vi "test_conv5.vi"() -> ()   [LabVIEW 2018]
uses:
  <vilib>/addons/Modulation/Digital/Channel Coding/MT Convolutional Encoder (Rate).vi
  <vilib>/addons/Modulation/Analog/support/mod_Set Error Source.vi
  <vilib>/addons/Modulation/Digital/Support/Common/Validators/mod_Validate Bit Stream.vi
  <vilib>/addons/Modulation/Digital/Channel Coding/Convolutional codes/mod_Convolutional encoder.vi
  <vilib>/addons/Modulation/Digital/Support/Common/Validators/mod_AWGN Validate.vi
  <vilib>/addons/Modulation/Digital/Impairments/subVIs/mod_createSeeds.vi
  <vilib>/addons/Modulation/Digital/Channel Coding/Convolutional codes/subVIs/mod_Generate encoder tap connections.vi
  <vilib>/addons/Modulation/Digital/Channel Coding/Convolutional codes/subVIs/mod_Perform convolutional encoding.vi
  <vilib>/addons/Modulation/Digital/Channel Coding/Block codes/subVIs/mod_Buffer block code info (I8).vi
  <vilib>/addons/Modulation/Digital/Channel Coding/Convolutional codes/subVIs/mod_Generate valid reset (convolutional, I8).vi
  <vilib>/addons/Modulation/Digital/Support/Common/Validators/mod_Validate Samples Per Symbol.vi
  <vilib>/addons/Modulation/Analog/support/Validators/mod_Validate Complex Waveform.vi
  <vilib>/addons/Modulation/Analog/support/Validators/mod_WFErrorHandler.vi
  <vilib>/addons/Modulation/Digital/Channel Coding/Convolutional codes/subVIs/mod_Select known generator matrix.vi
  <vilib>/addons/Modulation/Digital/Support/Common/Validators/mod_Validate Convolutional Encoder prms.vi
  <vilib>/addons/Modulation/Digital/Support/Common/Validators/mod_Generate Filter Coefficients Validate.vi
  <vilib>/addons/Modulation/Digital/General/subVIs/mod_Generate Filter Coefficients.vi
  <vilib>/addons/Modulation/Digital/General/MT Generate PSK System Parameters(M).vi
  <vilib>/addons/Modulation/Digital/General/subVIs/mod_Generate Bits PN Sequence.vi
  <vilib>/Analysis/1siggen.llb/Gaussian White Noise (obs 90).vi
  <vilib>/addons/Modulation/Digital/General/MT Apply Matched Filter (Generic).vi
  <vilib>/addons/Modulation/Digital/General/MT Map PSK Symbols to Bits.vi
  <vilib>/addons/Modulation/Digital/Channel Coding/MT Convolutional Decoder (Viterbi Hard Decision, Rate).vi
  <vilib>/addons/Modulation/niDMT.lvlib
panel:
  out "**** 5":i32
  out "**** 4":i32
  out "**** 3":i32
  out "**** 2":i32
  out "****":i32
  out "BER":dbl
  out "sigma2":string
  out "dec":i8[](array[numeric])
  out "message":i8[](array[numeric])
  out "IQ Constellation":T1(graph)
  out "BI  Dec":i8[](array[numeric])
  in  "Eb/N0":dbl=10.0 format="%.2f"
  in  "Traceback Depth (D)":i32=20
  in  "Constraint Length (K)":i32=3
  in  "Rate (k/n)":enum16{"1/2", "1/3", "1/4", "2/3", "3/4"}(ring)
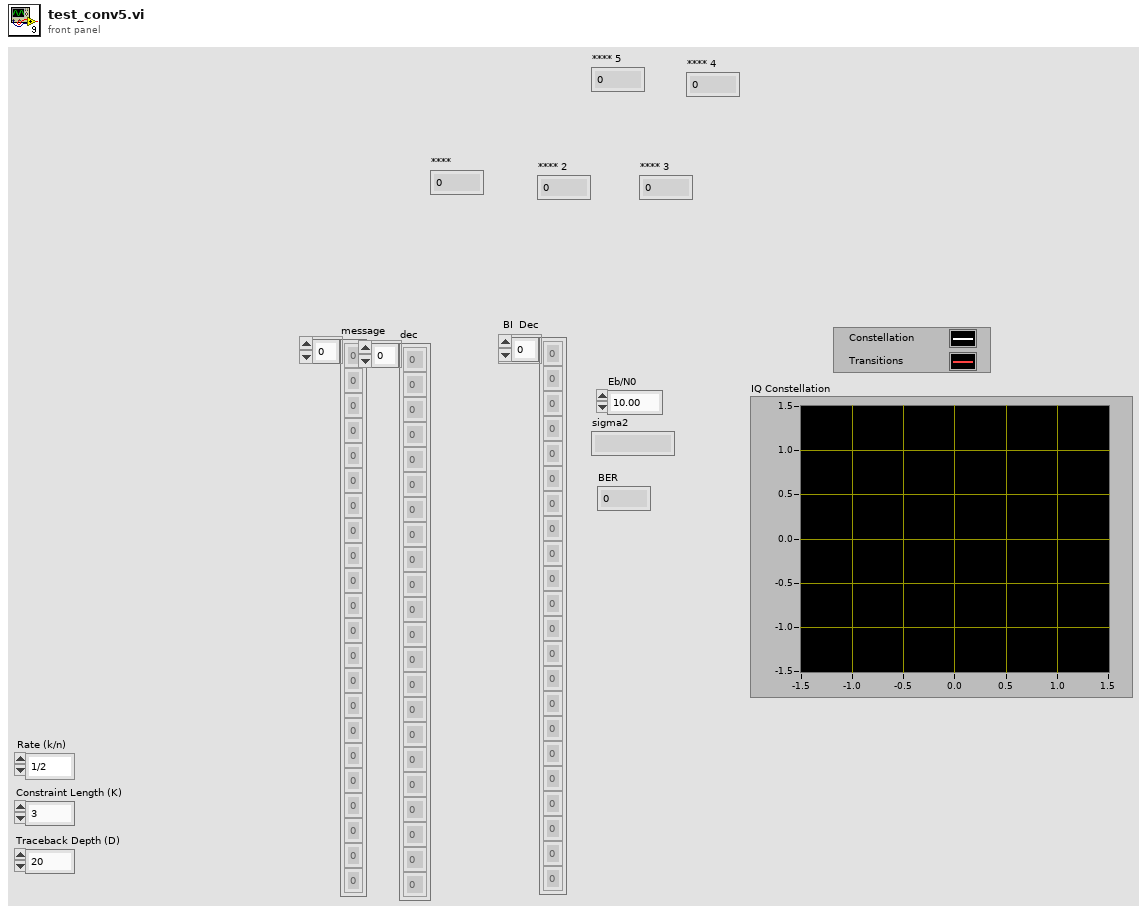
[diagram p1: front panel]
types:
  T1 = cluster{"Decimated Array":dbl[], "Decimated Array":dbl[]}[]
  T2 = enum16{"none", "Raised Cosine", "Root Raised Cos", "Gaussian"}
  T3 = cluster{"samples per symbol (16)":i32, "symbol map":cdb[], "differential PSK":enum16{"disable", "enable"}, "PSK type":u16}
  T4 = typedef "niAMT.lvlib/Complex Data Waveform.ctl" = cluster{"t0":dbl, "dt":dbl, "Y":cdb[]}
  T5 = cluster{"constellation":dbl[], "oversampled data":dbl[]}[]
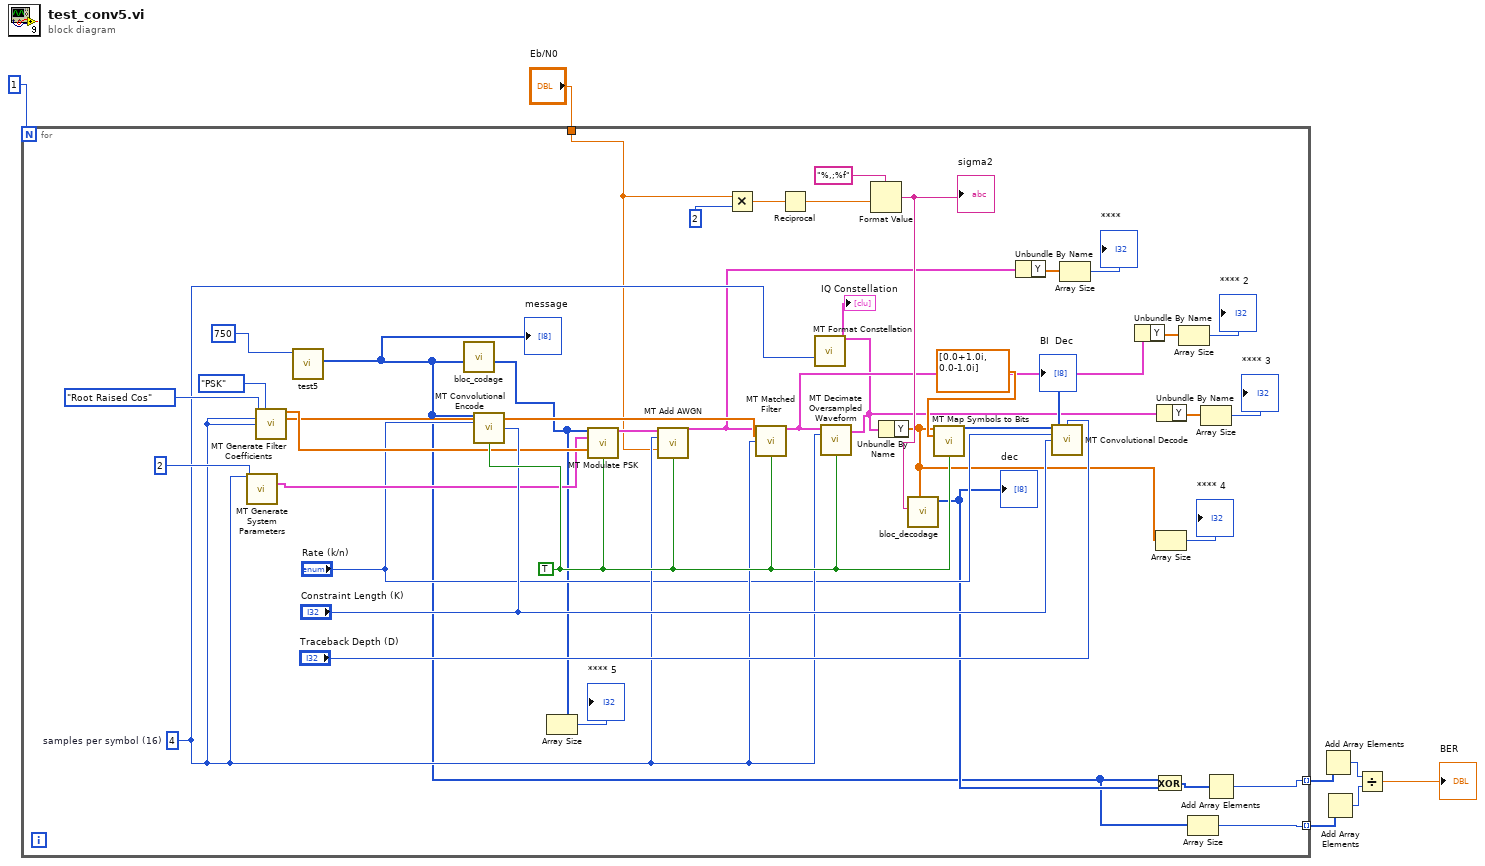
[diagram p0: block diagram]
diagram:
  n1 = for {
    N: 1 -> [_]
    tunnel: [w23] -> w5 mode=indexing
    tunnel: [w22] -> w4 mode=indexing
    tunnel: "Eb/N0" -> [w8]
    w35 = 4  # samples per symbol (16)
    w45 = TRUE ("reset? (T)")
    n2 = call-poly <vilib>:"MT Generate System Parameters.vi"("samples per symbol (16)"=w35, "M-PSK (4)"=2) -> ("PSK system parameters"=w34:T3)  [unwired: 11 in, 2 out]
    n3 = call <vilib>:"MT Generate Filter Coefficients.vi"("pulse shaping filter (none)"=T2."Root Raised Cos", "modulation type"=enum16{"FSK", "PSK", "QAM", "MSK", "PAM", "ASK"}."PSK", "pulse shaping samples per symbol (16)"=w35, "matched samples per symbol (16)"=w35) -> ("pulse shaping filter coefficients"=w37:dbl[], "matched filter coefficients"=w36:dbl[])  [unwired: 9 in, 1 out]
    n4 = call "test5.vi"("k"=750) -> ("output bit stream"=w24:i8[])  [unwired: 9 in, 1 out]
    "message" <- w24
    n5 = call "bloc_codage.vi"("Array in"=w24) -> ("output bit stream"=w9:i8[])  [unwired: 8 in, 2 out]
    n6 = call-poly <vilib>:"MT Convolutional Encode.vi"("input bit stream"=w24, "rate (k/n)"="Rate (k/n)", "constraint length (K)"="Constraint Length (K)", "reset? (T)"=w45) -> ()  [unwired: 9 in, 3 out]
    n7 = Array Size(array=w9) -> (size(s)=→"**** 5":i32)
    n8 = call <vilib>:"MT Modulate PSK.vi"("input bit stream"=w9, "PSK system parameters"=w34, "pulse shaping filter coefficients"=w37, "reset? (T)"=w45) -> ("output complex waveform"=w48:T4)  [unwired: 9 in, 2 out]
    n9 = call <vilib>:"MT Add AWGN.vi"("input complex waveform"=w48, "samples per symbol (16)"=w35, "Eb/N0 (10 dB)"=w8, "reset? (T)"=w45) -> ("output complex waveform"=w17:T4)  [unwired: 9 in, 2 out]
    n10 = Multiply(x=w8, y=2) -> (x*y=w30:dbl)
    n11 = call-poly <vilib>:"MT Matched Filter.vi"("input complex waveform"=w17, "matched filter coefficients"=w36, "samples per symbol (16)"=w35, "reset? (T)"=w45) -> ("output complex waveform"=w16:T4)  [unwired: 10 in, 1 out]
    n12 = Reciprocal(x=w30) -> (1/x=w27:dbl)
    n13 = call <vilib>:"MT Decimate Oversampled Waveform.vi"("input complex waveform"=w16, "decimation factor"=w35, "reset? (T)"=w45) -> ("output complex waveform"=w13:T4)  [unwired: 11 in, 1 out]
    n14 = call <vilib>:"MT Format Constellation.vi"("waveform"=w13, "samples per symbol"=w35) -> ("constellation graph"=→"IQ Constellation":T5)  [unwired: 12 in, 1 out]
    n15 = Format Value(format string="%,;%f", value (0)=w27) -> (output string=w28:string)  [unwired: 1 in]
    "sigma2" <- w28
    n16 = Unbundle By Name(w13) -> ("Y"=w11:cdb[])
    n17 = call "bloc_decodage.vi"("sigma2"=w28, "Array"=w11) -> ("output bit stream"=w26:i8[])  [unwired: 7 in, 2 out]
    "dec" <- w26
    n18 = call-poly <vilib>:"MT Map Symbols to Bits.vi"("symbols"=w11, "symbol map"=cdb[] [0.0+1.0i, 0.0-1.0i], "reset? (T)"=w45) -> ("output bit stream"=w43:i8[])  [unwired: 11 in, 1 out]
    n19 = Unbundle By Name(w17) -> ("Y"=w20:cdb[])
    n20 = call-poly <vilib>:"MT Convolutional Decode.vi"("input bit stream"=w43, "traceback depth (D)"="Traceback Depth (D)", "rate (k/n)"="Rate (k/n)", "constraint length (K)"="Constraint Length (K)") -> ("output bit stream"=→"BI  Dec":i8[])  [unwired: 9 in, 2 out]
    n21 = Array Size(array=w20) -> (size(s)=→"****":i32)
    n22 = Unbundle By Name(w16) -> ("Y"=w18:cdb[])
    n23 = Exclusive Or(1:w26, 2:w24) -> (0:w25:i8[])
    n24 = Array Size(array=w11) -> (size(s)=→"**** 4":i32)
    n25 = Unbundle By Name(w13) -> ("Y"=w14:cdb[])
    n26 = Array Size(array=w18) -> (size(s)=→"**** 2":i32)
    n27 = Array Size(array=w24) -> (size(s)=w22:i32)
    n28 = Array Size(array=w14) -> (size(s)=→"**** 3":i32)
    n29 = Add Array Elements(numeric array=w25) -> (sum=w23:i8)
  }
  n30 = Add Array Elements(numeric array=w5) -> (sum=w3:i8)
  n31 = Add Array Elements(numeric array=w4) -> (sum=w2:i32)
  n32 = Divide(x=w3, y=w2) -> (x/y=→"BER":dbl)
